vi "nonlinear_calibration_save(subVI).vi"(8 "error in (no error)":errorcluster, 9 "distanza fra marker":cluster{"X Step":sgl, "Y Step":sgl, "Unit":T2}={"X Step"=10.0, "Y Step"=10.0, "Unit"=enum."Millimeter"}, 10 "saving path Template Calibrazione":path=path "C:/Users/Dell/Desktop/Esame/LOAD/CalibrazioneMisura/calib-info.png", 11 "Image Src":T1) -> (0 "error out":errorcluster, 2 "Error Statistics":T4, 3 "Calibration Axis Info":T3={"Origin Pixel"={"X"=0.0, "Y"=0.0}, "Angle Relative to Horizontal (deg)"=0.0, "X Axis Pixel"={"X"=0.0, "Y"=0.0}, "Axis Reference"=1} {"X Axis Pixel"."Y" format="%.2f"; "X Axis Pixel"."X" format="%.2f"; "Axis Reference" items=["Direct", "Indirect"]; "Angle Relative to Horizontal (deg)" format="%.2f"; "Origin Pixel"."Y" format="%.2f"; "Origin Pixel"."X" format="%.2f"})   [LabVIEW 2020]
doc: "genera un template di calibrazione partenda da un immagine con il target in ingresso (image Src).\nsalva l'immagine di calibrazione al saving path."
uses:
  <vilib>/vision/Calibration.llb/Error Statistics.ctl
  <vilib>/vision/Image Controls.llb/IMAQ Image.ctl
  <vilib>/vision/Calibration.llb/Distortion Model.ctl
  <vilib>/vision/Calibration.llb/Distortion Model Types.ctl
  <vilib>/vision/NI_Vision_Development_Module.lvlib
panel:
  in  "stop":bool
  out "Error Map":sgl[][](array[numeric]) format="%.2f"
  out "Image":T1(plugin-control)
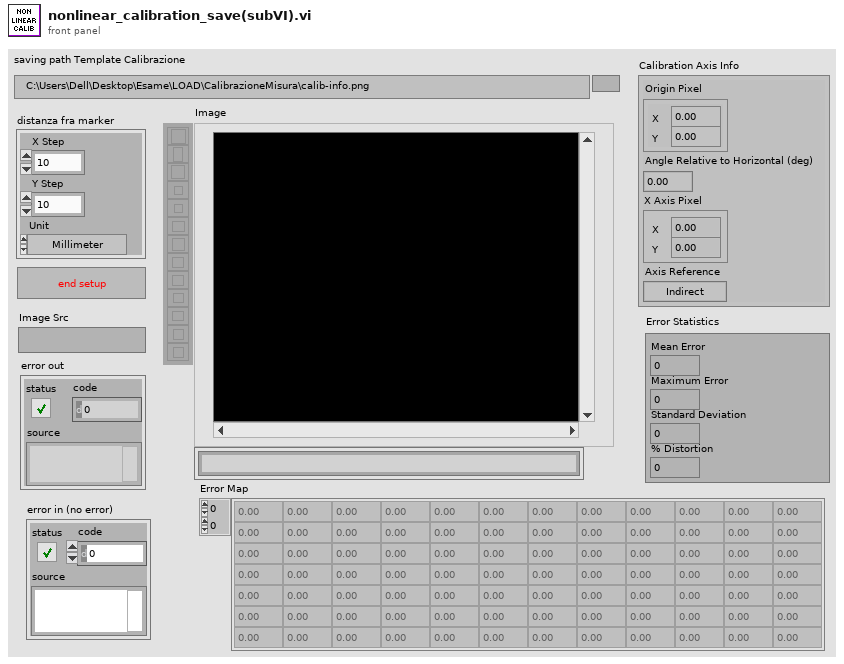
[diagram p1: front panel]
types:
  T1 = typedef "IMAQ Image.ctl" = refnum<image>
  T2 = typedef "Image Unit" = enum32{"Undefined", "Angström", "Micrometer", "Millimeter", "Centimeter", "Meter", "Kilometer", "Microinch", "Inch", "Feet", "Nautical miles", "Standard miles", "Steps"}
  T3 = cluster{"Origin Pixel":cluster{"X":sgl, "Y":sgl}, "Angle Relative to Horizontal (deg)":sgl, "X Axis Pixel":cluster{"X":sgl, "Y":sgl}, "Axis Reference":u32}
  T4 = typedef "Error Statistics.ctl" = cluster{"Mean Error":dbl, "Maximum Error":dbl, "Standard Deviation":dbl, "% Distortion":dbl}
  T5 = cluster{"Origin Pixel":cluster{"X":sgl, "Y":sgl}, "Angle Relative to Horizontal (deg)":sgl, "Axis Reference":u32}
  T6 = typedef "Distortion Model.ctl" = cluster{"Distortion Model":T7, "Polynomial Model Setup":cluster{"Radial Coefficient":u32, "Tangential Coefficients ":bool}}
  T7 = typedef "Distortion Model Types.ctl" = i32
  T8 = cluster{"Desired Font (Application)":enum16{"User-specified Font", "Application Font", "System Font", "Dialog Font"}, "[User-specified Font]":cluster{"Font Name":string, "Size":i16, "Strikeout?":bool, "Italic?":bool, "Underline?":bool, "Outline?":bool, "Shadow?":bool, "Bold?":bool, "Rotation Angle":dbl}, "Horizontal Alignment":i16, "Vertical Alignment":i16}
  T9 = typedef "Calibration Reference Points.ctl" = cluster{"Pixel Coordinates":cluster{"X":dbl, "Y":dbl}[], "Real World Coordinates":cluster{"X":dbl, "Y":dbl}[], "Unit":T2, "Image Size":cluster{"X":u32, "Y":u32}}
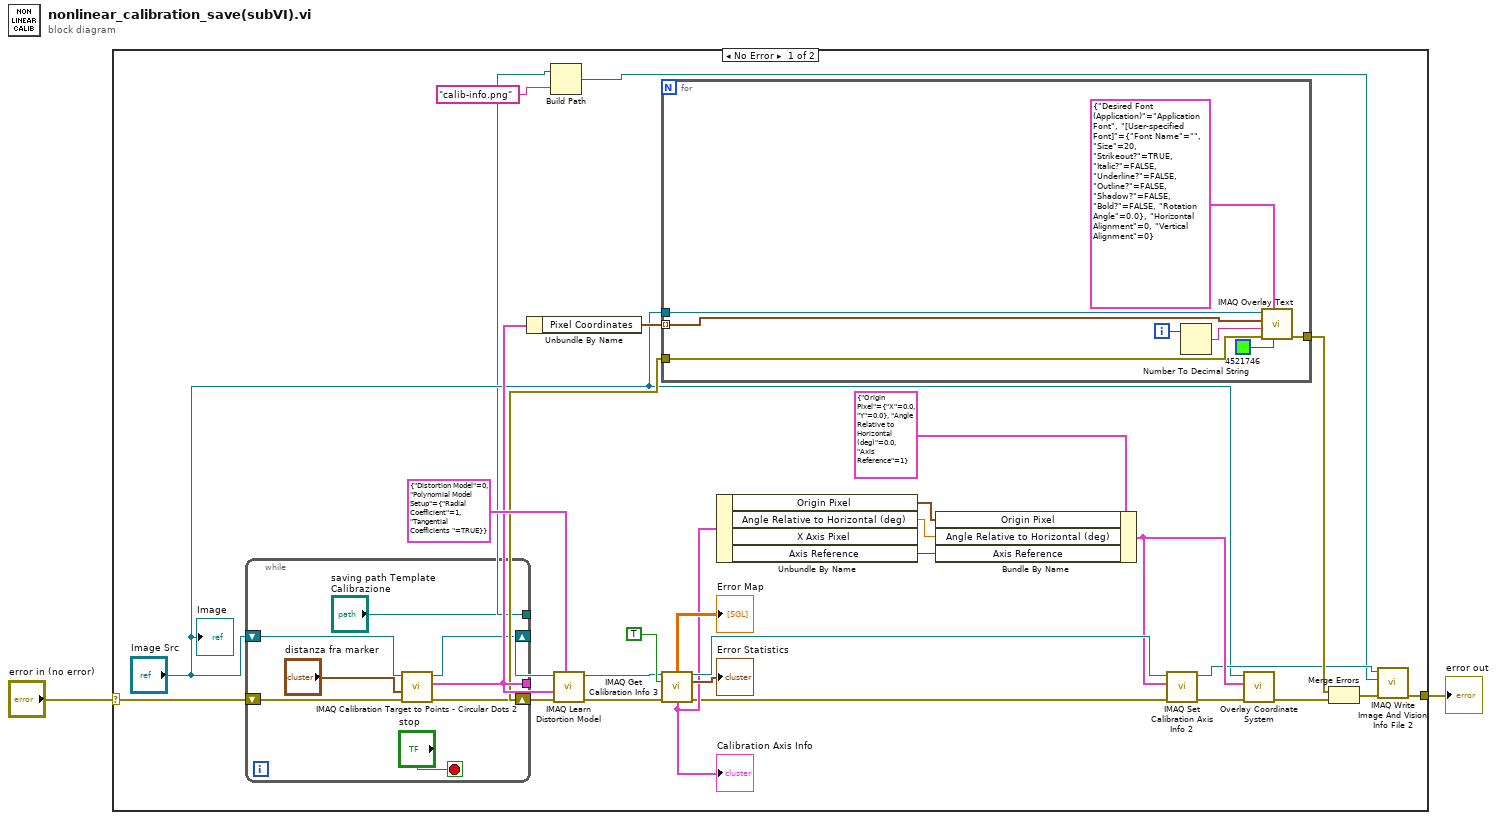
[diagram p0: block diagram]
diagram:
  n1 = case shown="No Error" "error in (no error)" {
    selector: "error in (no error)" -> [w7 w48]
    tunnel: [w8 w48] -> w2
    frame No Error {
      n2 = while {
        tunnel: [w37] -> w26
        shift-right: [w39] -> w31
        shift-left: "Image Src" -> [w35]
        shift-right: [w36] -> w25
        shift-left: w7 -> [w34]
        tunnel: ["saving path Template Calibrazione"] -> w5
        stop <- "stop" stop-if-true
        n3 = call "IMAQ Calibration Target to Points - Circular Dots 2"("error in (no error)"=w34, "Grid Descriptor"="distanza fra marker", "Target Image"=w35) -> ("error out"=w36:errorcluster, "Reference Points"=w37:T9, "Target Image (dup)"=w39:T1)  [unwired: 6 in]
      }
      n4 = Unbundle By Name(w26) -> ("Pixel Coordinates"=w23:cluster{"X":dbl, "Y":dbl}[])
      n5 = Build Path(base path=w5, name or relative path="calib-info.png") -> (appended path=w3:path)
      n6 = call "IMAQ Learn Distortion Model"("Distortion Model Setup"=T6 {"Distortion Model"=0, "Polynomial Model Setup"={"Radial Coefficient"=1, "Tangential Coefficients "=TRUE}}, "error in (no error)"=w25, "Reference Points"=w26, "Calibration Template Image"=w31) -> ("error out"=w12:errorcluster, "Calibration Template Image Out"=w11:T1)  [unwired: 6 in]
      n7 = for {
        tunnel: w25 -> [w47]
        tunnel: [w46] -> w24
        tunnel: w23 -> [w45] mode=indexing
        tunnel: "Image Src" -> [w40]
        i -> [w44]
        n8 = Number To Decimal String(number=w44) -> (decimal integer string=w43:string)  [unwired: 1 in]
        n9 = call "IMAQ Overlay Text"("Text Color (black)"=u32 4521746, "Font, Size & Style"=T8 {"Desired Font (Application)"=enum."Application Font", "[User-specified Font]"={"Font Name"="", "Size"=20, "Strikeout?"=TRUE, "Italic?"=FALSE, "Underline?"=FALSE, "Outline?"=FALSE, "Shadow?"=FALSE, "Bold?"=FALSE, "Rotation Angle"=0.0}, "Horizontal Alignment"=0, "Vertical Alignment"=0}, "error in (no error)"=w47, "String"=w43, "Origin"=w45, "Image"=w40) -> ("error out"=w46:errorcluster)  [unwired: 4 in, 1 out]
      }
      n10 = call "IMAQ Get Calibration Info 3"("Calibration Template Image"=w11, "Return Error Information (False)"=TRUE, "error in (no error)"=w12) -> ("Error Map"=→"Error Map":sgl[][], "Calibration Template Image (duplicate)"=w22:T1, "Error Statistics"=→"Error Statistics":T4, "Calibration Axis Info"=w21:T3, "error out"=w16:errorcluster)  [unwired: 4 in, 4 out]
      "Calibration Axis Info" <- w21
      n11 = Unbundle By Name(w21) -> ("Origin Pixel"=w19:cluster{"X":sgl, "Y":sgl}, "Angle Relative to Horizontal (deg)"=w18:sgl, "Axis Reference"=w17:u32)  [unwired: 1 out]
      n12 = Bundle By Name(cluster=T5 {"Origin Pixel"={"X"=0.0, "Y"=0.0}, "Angle Relative to Horizontal (deg)"=0.0, "Axis Reference"=1} ("Calibration Axis Info 2"), "Origin Pixel"=w19, "Angle Relative to Horizontal (deg)"=w18, "Axis Reference"=w17) -> (w15:T5)
      n13 = call-poly "IMAQ Set Calibration Axis Info 2"("error in (no error)"=w16, "Calibration Axis Info"=w15, "Calibration Template Image In"=w22) -> ("error out"=w14:errorcluster, "Calibration Template Image Out"=w10:T1)  [unwired: 7 in]
      n14 = call "Overlay Coordinate System.vi"("error in"=w14, "Calibration Axis Info"=w15, "Image"="Image Src") -> ("error out"=w13:errorcluster)  [unwired: 7 in, 1 out]
      n15 = Merge Errors(w24, w13) -> (w9:errorcluster)
      n16 = call "IMAQ Write Image And Vision Info File 2"("error in (no error)"=w9, "File Path"=w3, "Image"=w10) -> ("error out"=w8:errorcluster)  [unwired: 7 in, 1 out]
      "Image" <- "Image Src"
    }
    frame Error {
    }
  }
  "error out" <- w2
